vi "FindLineAndOverwrite_Double.vi"(0 "Exposure path":path, 5 "Name":string, 7 "Index":u32, 9 "Exposure":dbl, 11 "error in (no error)":errorcluster) -> (15 "error out":errorcluster)   [LabVIEW 2014]
panel:
  out "match substring":string
  out "Input String":string
  out "Output string":string
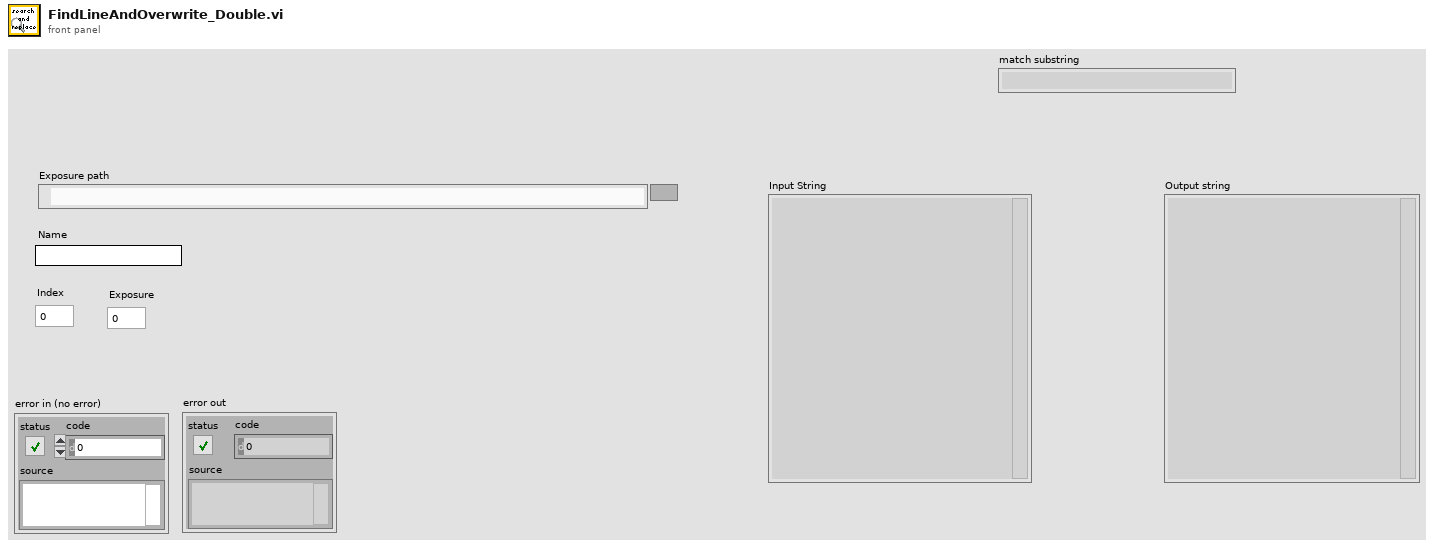
[diagram p1: front panel]
types:
  T1 = enum16{"open", "replace", "create", "open or create", "replace or create", "replace or create with confirmation"}
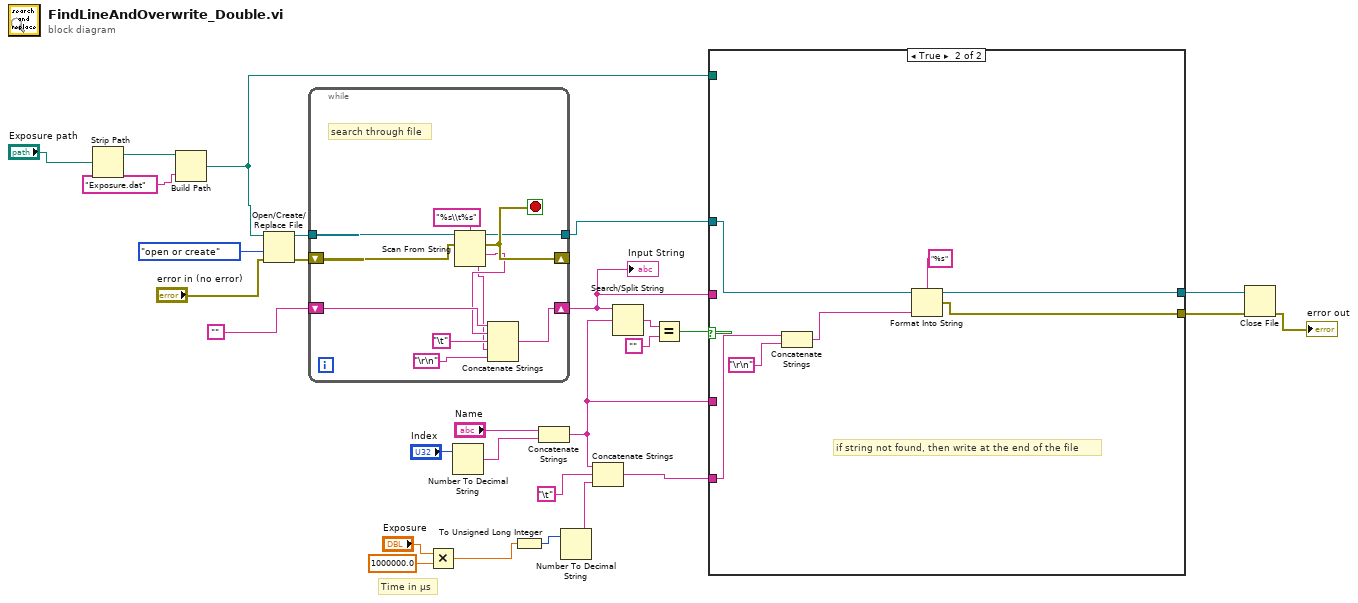
[diagram p0: block diagram]
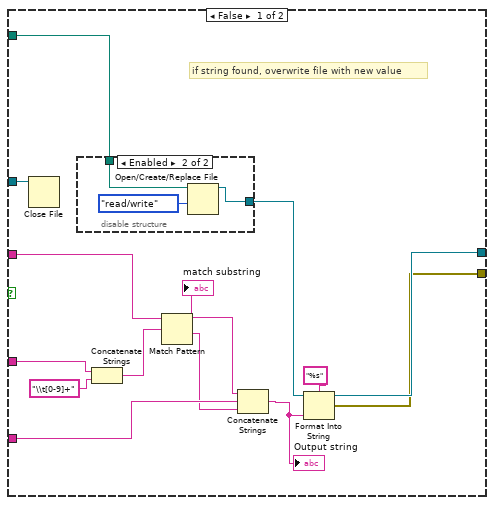
[diagram p2: hidden frame]
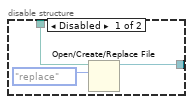
[diagram p3: hidden frame]
diagram:
  # "Time in µs"
  n1 = Strip Path(path="Exposure path") -> (stripped path=w9:path)  [unwired: 1 out]
  n2 = Build Path(base path=w9, name or relative path="Exposure.dat") -> (appended path=w6:path)
  n3 = Open/Create/Replace File(file path (use dialog)=w6, error in="error in (no error)", operation (0:open)=T1."open or create") -> (refnum out=w22:refnum<file>, error out=w21:errorcluster)  [unwired: 3 in, 1 out]
  n4 = while {
    tunnel: w22 -> [w38]
    shift-right: [w36] -> _
    shift-left: w21 -> [w37]
    shift-right: [w35] -> w13
    shift-left: "" -> [w33]
    tunnel: [w34] -> w16
    stop <- w36 stop-if-true
    # "search through file"
    n5 = Scan From String("%s\\t%s" ("format string"), w38, w37) -> (w34:refnum<file>, w36:errorcluster, output 1=w32:string, output 2=w30:string)  [unwired: 2 in]
    n6 = Concatenate Strings(w33, w32, "\t", w30, "\r\n") -> (w35:string)
  }
  "Input String" <- w13
  n7 = Multiply(x="Exposure", y=1000000.0) -> (x*y=w1:dbl)
  n8 = Number To Decimal String(number="Index") -> (decimal integer string=w27:string)  [unwired: 1 in]
  n9 = To Unsigned Long Integer(number=w1) -> (unsigned 32bit integer=w5:u32)
  n10 = Concatenate Strings("Name", w27) -> (w10:string)
  n11 = Number To Decimal String(number=w5) -> (decimal integer string=w4:string)  [unwired: 1 in]
  n12 = Concatenate Strings(w10, "\t", w4) -> (w14:string)
  n13 = Search/Split String(string=w13, search string/char (-)=w10) -> (match + rest of string=w19:string)  [unwired: 1 in, 2 out]
  n14 = Equal?(x=w19, y="") -> (x = y?=w17:bool)
  n15 = case shown="True" w17 {
    tunnel: w16 -> [w54 w66]
    tunnel: w14 -> [w49 w63]
    tunnel: w13 -> [w53 _]
    tunnel: [w45 w65] -> w12
    tunnel: [w44 w64] -> w11
    tunnel: w10 -> [w52 _]
    tunnel: w6 -> [w47 _]
    frame False {
      # "if string found, overwrite file with new value"
      n16 = Close File(refnum=w54) -> ()  [unwired: 1 in, 2 out]
      n17 = disable-structure shown="Enabled" {
        disable-tunnel: w47 -> [w56 w59]
        disable-tunnel: [w55 w58] -> w46
        frame Disabled {
          n18 = Open/Create/Replace File(file path (use dialog)=w56, operation (0:open)=T1."replace") -> (refnum out=w55:refnum<file>)  [unwired: 4 in, 2 out]
        }
        frame Enabled {
          n19 = Open/Create/Replace File(file path (use dialog)=w59, access (0:read/write)=enum16{"read/write", "read-only", "write-only"}."read/write") -> (refnum out=w58:refnum<file>)  [unwired: 4 in, 2 out]
        }
      }
      n20 = Concatenate Strings(w52, "\\t[0-9]+" ("regular expression")) -> (w51:string)
      n21 = Match Pattern(string=w53, regular expression=w51) -> (before substring=w50:string, match substring=→"match substring":string, after substring=w48:string)  [unwired: 1 in, 1 out]
      n22 = Concatenate Strings(w50, w49, w48) -> (w40:string)
      "Output string" <- w40
      n23 = Format Into String(format string="%s" ("format (%.3f)"), initial string=w46, w40) -> (resulting string=w45:refnum<file>, error out=w44:errorcluster)  [unwired: 1 in]
    }
    frame True {
      # "if string not found, then write at the end of the file"
      n24 = Concatenate Strings(w63, "\r\n") -> (w61:string)
      n25 = Format Into String(format string="%s" ("format (%.3f)"), initial string=w66, w61) -> (resulting string=w65:refnum<file>, error out=w64:errorcluster)  [unwired: 1 in]
    }
  }
  n26 = Close File(refnum=w12, error in=w11) -> (error out=→"error out":errorcluster)  [unwired: 1 out]
